vi "Physics_Engine_Core.vi"(0 "Design Constants":T6={"P_amb (psia)"=0.125, "T_in (Deg F)"=14.7, "R_air (ft*lbf)/(lbm*R)"=530.0, "g_c (lbm*ft)/(lbf*s^2)"=53.35, "specific heat ratio"=32.17, "Viscousity (lbm)/(ft*s)"=1.4, "Cd"=0.95, "Mass Flow (lbm/min) vs. Pressure Drop (inH2O) - Real Data"=[[0.5, 0.015], [1.0, 0.062], [1.5, 0.141], [2.0, 0.252], [2.5, 0.395], [3.5, 0.778]]} {"Mass Flow (lbm/min) vs. Pressure Drop (inH2O) - Real Data" format="%_3g"; "P_amb (psia)" format="%#_4g"}, 1 "Calibration Data":T8, 4 "Design Tuners":T7 {"OAR" items=["0.92"=0.92, "0.93"=0.93, "0.94"=0.94, "0.95"=0.95, "0.96"=0.96]; "D_h (in)" items=["0.0625"=0.0625, "0.125"=0.125, "0.250"=0.25]; "Pipe_Diameter (in)" min=0.1 max=6.0 scale=0.0..6.0 scale format="%#_3g"; "Length (in)" min=0.1 max=5.0 scale=0.0..6.0 scale format="%#_3g"; "Outlet Diameter (in)" min=0.1 max=5.0 scale=0.0..5.0 scale format="%#_3g"; "Inlet Diameter (in)" min=0.1 max=5.0 scale=0.0..5.0}, 5 "error in (no error)":errorcluster, 6 "Enum":T5) -> (14 "empirical curve":T3, 15 "total curve":T2, 16 "tap curve":T1, 17 "outcome":cluster{"pass/fail":dbl[], "error_pct":dbl[]}, 18 "parameters_output":T4, 19 "error out":errorcluster)   [LabVIEW 2025, in "Acquisition.lvlib"]
uses:
  Acquisition/Acquisition.lvlib
  controls/Calibration_Data.ctl
  controls/Tuners.ctl
  controls/Constants.ctl
  controls/Mode Enum.ctl
panel:
  out "Re_c":dbl[](array[numeric])
  # "Empirical Flow Path Data"
  # "Mass Flow\n (lbm/min)"
  # "Pressure Drop \n    (inH2O)"
  # "Honeycomb Parameters"
  # "Orifice Parameters"
  # "Pipe Parameters"
  # "AIRFLOW SIMULATOR"
  # "Mass_flowrate"
  # "Pipe_Diameter"
  # "Outlet_Diameter"
  # "Inlet_Diameter"
  # "Honeycomb_Length"
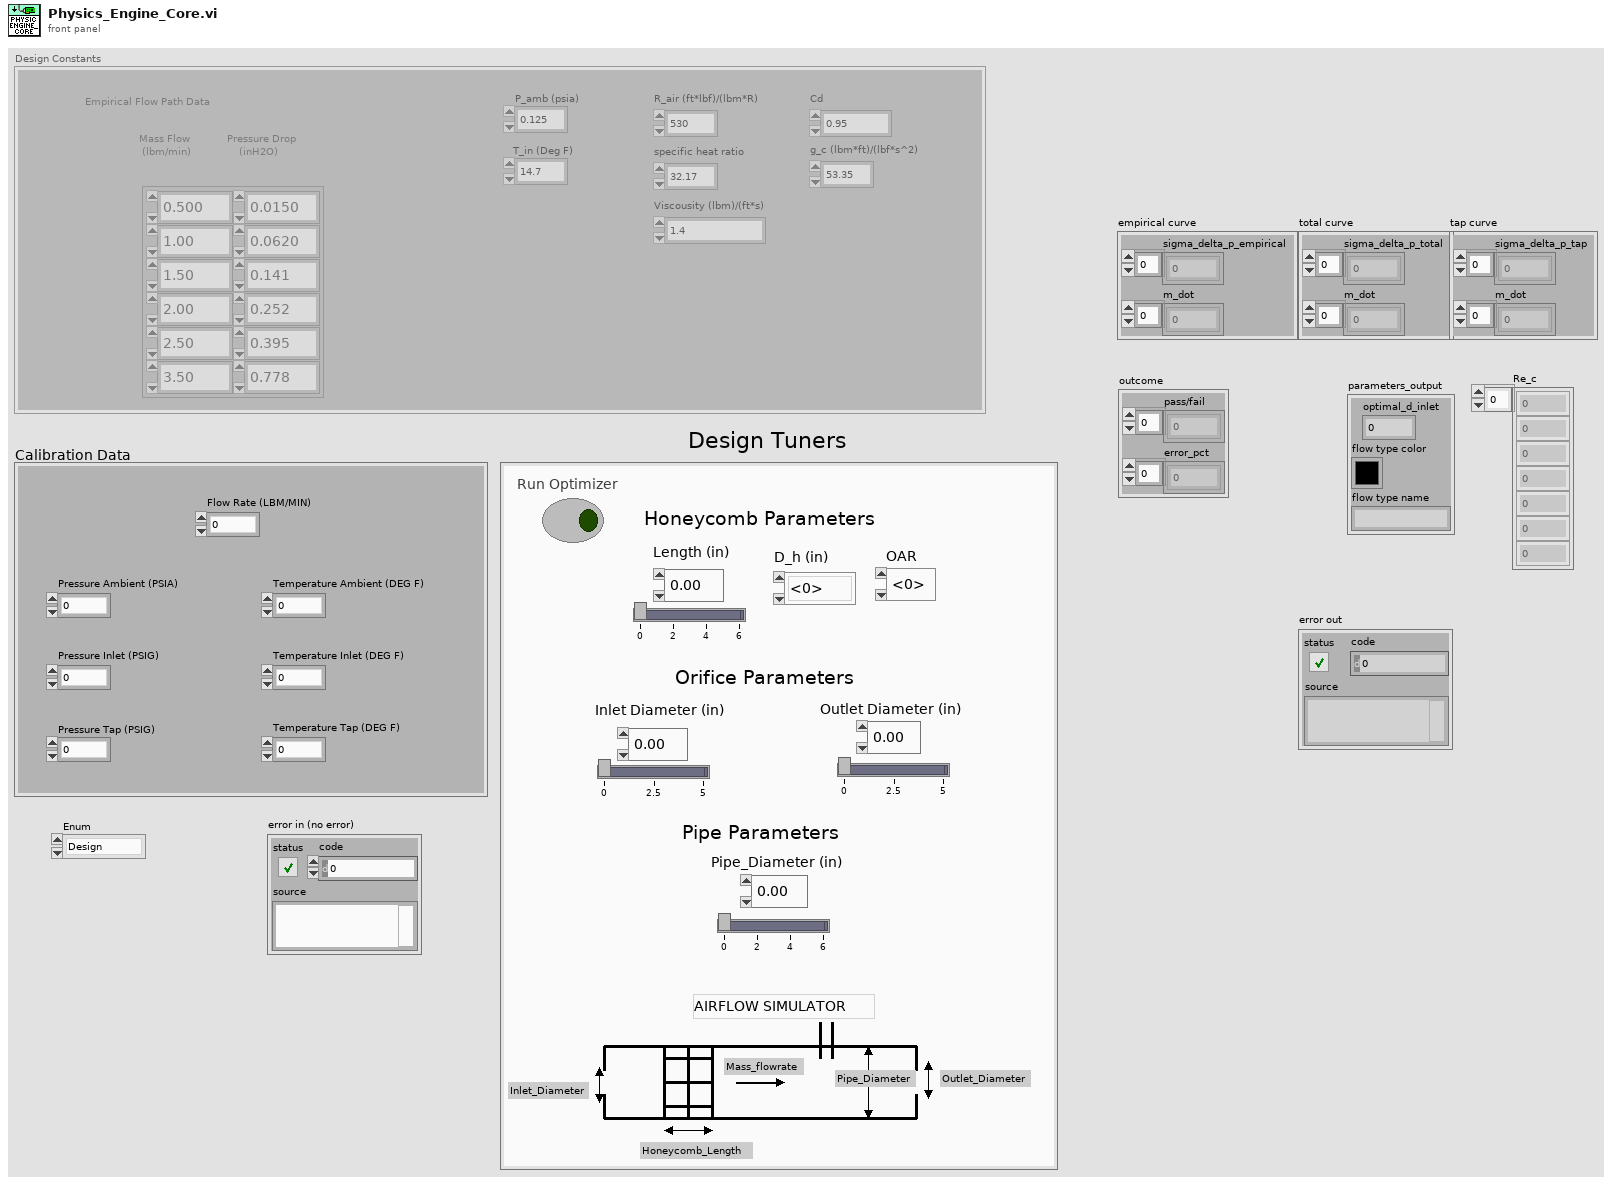
[diagram p1: front panel]
types:
  T1 = cluster{"sigma_delta_p_tap":dbl[], "m_dot":dbl[]}
  T2 = cluster{"sigma_delta_p_total":dbl[], "m_dot":dbl[]}
  T3 = cluster{"sigma_delta_p_empirical":dbl[], "m_dot":dbl[]}
  T4 = cluster{"optimal_d_inlet":dbl, "flow type color":u32, "flow type name":string}
  T5 = typedef "Mode Enum.ctl" = enum16{"Design", "Calibration"}
  T6 = typedef "Constants.ctl" = cluster{"P_amb (psia)":dbl, "T_in (Deg F)":dbl, "R_air (ft*lbf)/(lbm*R)":dbl, "g_c (lbm*ft)/(lbf*s^2)":dbl, "specific heat ratio":dbl, "Viscousity (lbm)/(ft*s)":dbl, "Cd":dbl, "Mass Flow (lbm/min) vs. Pressure Drop (inH2O) - Real Data":dbl[][]}
  T7 = typedef "Tuners.ctl" = cluster{"Inlet Diameter (in)":dbl, "Outlet Diameter (in)":dbl, "Length (in)":dbl, "Pipe_Diameter (in)":dbl, "D_h (in)":dbl, "OAR":dbl, "Run Optimizer":bool}
  T8 = typedef "Calibration_Data.ctl" = cluster{"Flow Rate (LBM/MIN)":dbl, "Pressure Ambient (PSIA)":dbl, "Pressure Inlet (PSIG)":dbl, "Pressure Tap (PSIG)":dbl, "Temperature Ambient (DEG F)":dbl, "Temperature Inlet (DEG F)":dbl, "Temperature Tap (DEG F)":dbl}
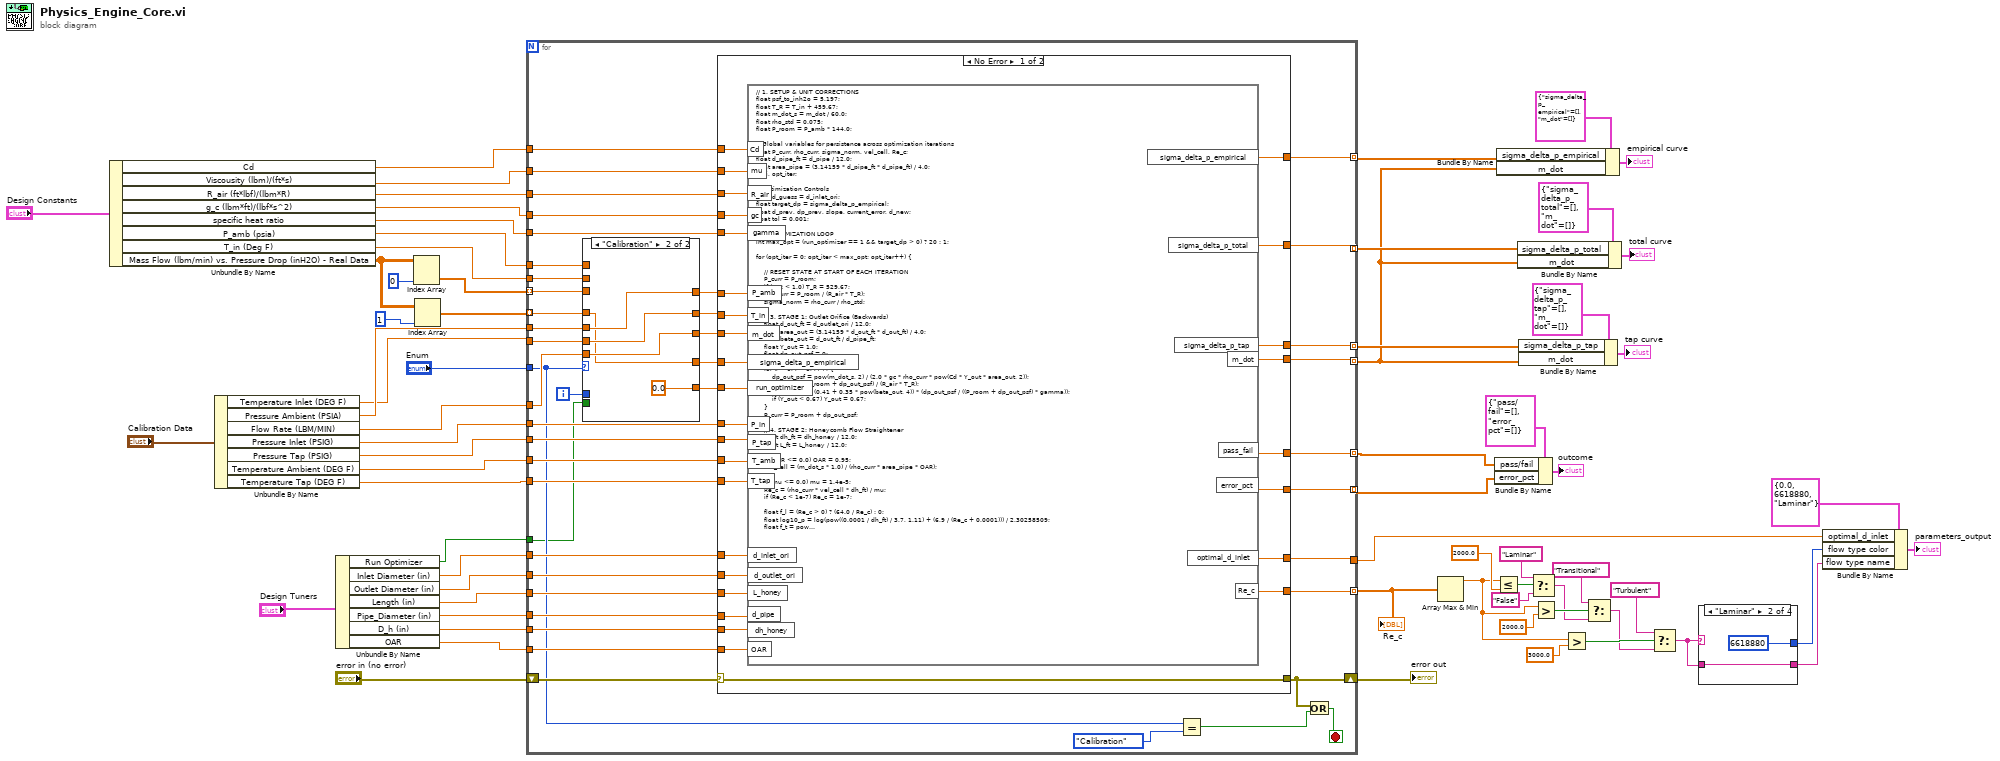
[diagram p0: block diagram]
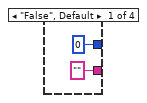
[diagram p2: hidden frame]
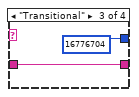
[diagram p3: hidden frame]
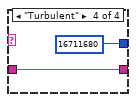
[diagram p4: hidden frame]
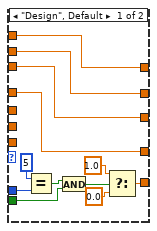
[diagram p5: hidden frame]
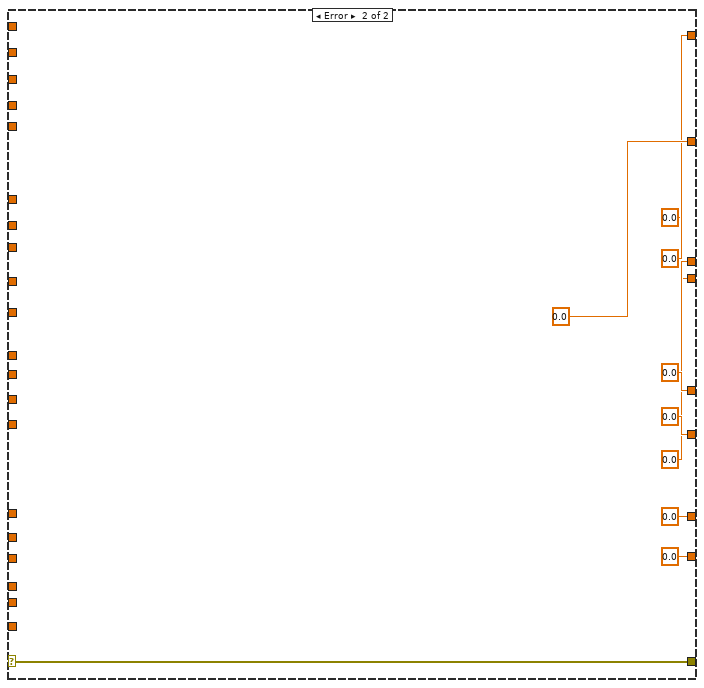
[diagram p6: hidden frame]
diagram:
  n1 = Unbundle By Name("Design Constants") -> ("Cd"=w46:dbl, "Viscousity (lbm)/(ft*s)"=w47:dbl, "R_air (ft*lbf)/(lbm*R)"=w48:dbl, "g_c (lbm*ft)/(lbf*s^2)"=w49:dbl, "specific heat ratio"=w50:dbl, "P_amb (psia)"=w41:dbl, "T_in (Deg F)"=w43:dbl, "Mass Flow (lbm/min) vs. Pressure Drop (inH2O) - Real Data"=w37:dbl[][])
  n2 = Unbundle By Name("Calibration Data") -> ("Temperature Inlet (DEG F)"=w42:dbl, "Pressure Ambient (PSIA)"=w44:dbl, "Flow Rate (LBM/MIN)"=w63:dbl, "Pressure Inlet (PSIG)"=w62:dbl, "Pressure Tap (PSIG)"=w61:dbl, "Temperature Ambient (DEG F)"=w60:dbl, "Temperature Tap (DEG F)"=w59:dbl)
  n3 = Unbundle By Name("Design Tuners") -> ("Run Optimizer"=w35:bool, "Inlet Diameter (in)"=w57:dbl, "Outlet Diameter (in)"=w56:dbl, "Length (in)"=w52:dbl, "Pipe_Diameter (in)"=w53:dbl, "D_h (in)"=w55:dbl, "OAR"=w54:dbl)
  n4 = Index Array(array=w37, index (col)=0) -> (element=w39:dbl[])  [unwired: 1 in]
  n5 = Index Array(array=w37, index (col)=1) -> (element=w36:dbl[])  [unwired: 1 in]
  n6 = for {
    tunnel: w63 -> [w82]
    tunnel: w62 -> [w108]
    tunnel: w61 -> [w107]
    tunnel: w60 -> [w106]
    tunnel: w59 -> [w105]
    tunnel: w57 -> [w104]
    tunnel: w56 -> [w103]
    tunnel: w55 -> [w102]
    tunnel: w54 -> [w101]
    tunnel: w53 -> [w100]
    tunnel: w52 -> [w99]
    tunnel: w50 -> [w98]
    tunnel: w49 -> [w97]
    tunnel: w48 -> [w96]
    tunnel: w47 -> [w95]
    tunnel: w46 -> [w94]
    tunnel: [w93] -> w8 mode=indexing
    shift-right: [w77] -> w65
    shift-left: "error in (no error)" -> [w109]
    tunnel: "Enum" -> [w78]
    tunnel: w44 -> [w92]
    tunnel: w43 -> [w91]
    tunnel: w42 -> [w90]
    tunnel: w41 -> [w89]
    tunnel: w39 -> [w88] mode=indexing
    tunnel: w36 -> [w84] mode=indexing
    tunnel: [w81] -> w11 mode=indexing
    tunnel: [w80] -> w13 mode=indexing
    tunnel: [w74] -> w5 mode=indexing
    tunnel: [w73] -> w19
    tunnel: w35 -> [w70]
    tunnel: [w69] -> w20 mode=indexing
    tunnel: [w68] -> w9 mode=indexing
    tunnel: [w67] -> w4 mode=indexing
    i -> [w72]
    stop <- w75 stop-if-true
    n7 = case shown="\"Calibration\"" w78 {
      tunnel: w92 -> [_ w126]
      tunnel: [w121 w126] -> w87
      tunnel: w91 -> [w120 _]
      tunnel: w90 -> [_ w125]
      tunnel: [w120 w125] -> w86
      tunnel: w89 -> [w121 _]
      tunnel: w88 -> [w119 _]
      tunnel: [w119 w124] -> w85
      tunnel: w84 -> [w118 w123]
      tunnel: [w118 w123] -> w83
      tunnel: w82 -> [_ w124]
      tunnel: w72 -> [w111 _]
      tunnel: [w116 0.0 ("f")] -> w71
      tunnel: w70 -> [w110 _]
      frame "Design", Default {
        n8 = Equal?(x=5 ("y"), y=w111) -> (x = y?=w114:bool)
        n9 = And(x=w114, y=w110) -> (x .and. y?=w113:bool)
        n10 = Select(t=1.0, s=w113, f=0.0) -> (s? t:f=w116:dbl)
      }
      frame "Calibration" {
      }
    }
    n11 = case shown="No Error" w109 {
      selector: w109 -> [w143 w164]
      tunnel: [w143 w164] -> w77
      tunnel: w87 -> [w155 _]
      tunnel: w85 -> [w154 _]
      tunnel: w108 -> [w153 _]
      tunnel: w107 -> [w152 _]
      tunnel: w106 -> [w151 _]
      tunnel: w105 -> [w150 _]
      tunnel: w104 -> [w149 _]
      tunnel: w103 -> [w148 _]
      tunnel: w102 -> [w147 _]
      tunnel: w101 -> [w146 _]
      tunnel: w100 -> [w145 _]
      tunnel: w99 -> [w144 _]
      tunnel: w86 -> [w142 _]
      tunnel: w98 -> [w141 _]
      tunnel: w97 -> [w140 _]
      tunnel: w96 -> [w139 _]
      tunnel: w95 -> [w138 _]
      tunnel: w94 -> [w137 _]
      tunnel: [w136 0.0 ("sigma_delta_p")] -> w93
      tunnel: w83 -> [w135 _]
      tunnel: [w134 0.0 ("pass_fail")] -> w81
      tunnel: [w133 0.0 ("error_pct")] -> w80
      tunnel: [w132 0.0 ("sigma_delta_p_tap")] -> w74
      tunnel: [w131 0.0 ("optimal_d_inlet")] -> w73
      tunnel: w71 -> [w130 _]
      tunnel: [w129 0.0] -> w69
      tunnel: [w128 0.0 ("sigma_delta_p_empirical")] -> w68
      tunnel: [w127 0.0 ("m_dot")] -> w67
      frame No Error {
        n12 = formula code="// 1. SETUP & UNIT CORRECTIONS\nfloat psf_to_inh2o = 5.197;\nfloat T_R = T_in + 459.67;\nfloat m_dot_s = m_dot / 60.0;\nfloat rho_std = 0.075;\nfloat P_room = P_amb * 144.0;\n\n// Global variables for persistence across optimization iterations\nfloat P_curr, rho_curr, sigma_norm, vel_cell, Re_c; \nfloat d_pipe_ft = d_pipe / 12.0;\nfloat area_pipe = (3.14159 * d_pipe_ft * d_pipe_ft) / 4.0;\nint i, opt_iter;\n\n// Optimization Controls\nfloat d_guess = d_inlet_ori;\nfloat target_dp = sigma_delta_p_empirical;\nfloat d_prev, dp_prev, slope, current_error, d_new;\nfloat tol = 0.001; \n\n// 2. OPTIMIZATION LOOP\nint max_opt = (run_optimizer == 1 && target_dp > 0) ? 20 : 1;\n\nfor (opt_iter = 0; opt_iter < max_opt; opt_iter++) {\n    \n    // RESET STATE AT START OF EACH ITERATION\n    P_curr = P_room;\n    if (T_R < 1.0) T_R = 529.67; \n    rho_curr = P_room / (R_air * T_R);\n    sigma_norm = rho_curr / rho_std;\n\n    // 3. STAGE 1: Outlet Orifice (Backwards)\n    float d_out_ft = d_outlet_ori / 12.0;\n    float area_out = (3.14159 * d_out_ft * d_out_ft) / 4.0;\n    float beta_out = d_out_ft / d_pipe_ft;\n    float Y_out = 1.0;\n    float dp_out_psf = 0;\n\n    for (i = 0; i < 8; i++) {\n        dp_out_psf = pow(m_dot_s, 2) / (2.0 * gc * rho_curr * pow(Cd * Y_out * area_out, 2));\n        rho_curr = (P_room + dp_out_psf) / (R_air * T_R);\n        Y_out = 1.0 - (0.41 + 0.35 * pow(beta_out, 4)) * (dp_out_psf / ((P_room + dp_out_psf) * gamma));\n        if (Y_out < 0.67) Y_out = 0.67;\n    }\n    P_curr = P_room + dp_out_psf;\n\n    // 4. STAGE 2: Honeycomb Flow Straightener\n    float dh_ft = dh_honey / 12.0;\n    float L_ft = L_honey / 12.0;\n    \n    if (OAR <= 0.0) OAR = 0.95; \n    vel_cell = (m_dot_s * 1.0) / (rho_curr * area_pipe * OAR);\n\n    if (mu <= 0.0) mu = 1.4e-5;\n    Re_c = (rho_curr * vel_cell * dh_ft) / mu;\n    if (Re_c < 1e-7) Re_c = 1e-7; \n\n    float f_l = (Re_c > 0) ? (64.0 / Re_c) : 0;\n    float log10_p = log(pow((0.0001 / dh_ft) / 3.7, 1.11) + (6.9 / (Re_c + 0.0001))) / 2.30258509;\n    float f_t = pow(1.0 / (-1.8 * log10_p), 2);\n    float f_h = (Re_c < 2000) ? f_l : (Re_c > 3000 ? f_t : (f_l + f_t)/2.0);\n\n    P_curr += f_h * (L_ft / dh_ft) * (rho_curr * vel_cell * vel_cell) / (2.0 * gc);\n    rho_curr = P_curr / (R_air * T_R);\n    \n    // CAPTURE TAP PRESSURE (Tap-to-Exit)\n    sigma_delta_p_tap = ((P_curr - P_room) / psf_to_inh2o) * sigma_norm;\n\n    // 5. STAGE 3: Inlet Orifice (Variable for Optimization)\n    float d_in_ft = d_guess / 12.0;\n    float area_in = (3.14159 * d_in_ft * d_in_ft) / 4.0;\n    float beta_in = d_in_ft / d_pipe_ft;\n    float Y_in = 1.0;\n    float dp_in_psf = 0;\n\n    for (i = 0; i < 8; i++) {\n        dp_in_psf = pow(m_dot_s, 2) / (2.0 * gc * rho_curr * pow(Cd * Y_in * area_in, 2));\n        rho_curr = (P_curr + dp_in_psf) / (R_air * T_R);\n        Y_in = 1.0 - (0.41 + 0.35 * pow(beta_in, 4)) * (dp_in_psf / ((P_curr + dp_in_psf) * gamma));\n        if (Y_in < 0.67) Y_in = 0.67;\n    }\n\n    // 6. TOTAL CALCULATION (Inlet-to-Exit)\n    sigma_delta_p_total = ((P_curr + dp_in_psf - P_room) / psf_to_inh2o) * sigma_norm;\n\n    // OPTIMIZER STEP (Matches Total Pressure to Empirical Target)\n    if (run_optimizer == 1) {\n        current_error = sigma_delta_p_total - target_dp;\n        if (abs(current_error) < tol) break; \n\n        if (opt_iter == 0) {\n            d_prev = d_guess;\n            dp_prev = sigma_delta_p_total;\n            d_guess += (d_guess * 0.01); \n        } else {\n            slope = (sigma_delta_p_total - dp_prev) / (d_guess - d_prev);\n            d_prev = d_guess;\n            dp_prev = sigma_delta_p_total;\n            d_new = d_guess - 0.8 * (current_error / slope);\n            d_guess = d_new;\n        }\n        \n        if (d_guess < 0.2) d_guess = 0.2;\n        if (d_guess > (d_pipe * 0.95)) d_guess = d_pipe * 0.95;\n    }\n}\n\n// 7. FINAL OUTPUTS\noptimal_d_inlet = (d_guess != d_guess) ? d_inlet_ori : d_guess;\n\nif (target_dp != 0) {\n    error_pct = ((sigma_delta_p_total - target_dp) / target_dp) * 100.0;\n} else {\n    error_pct = 0;\n}\n\npass_fail = (abs(error_pct) <= 2.0) ? 1 : 0;"("P_amb"=w155, "m_dot"=w154, "P_in"=w153, "P_tap"=w152, "T_amb"=w151, "T_in"=w142, "T_tap"=w150, "d_inlet_ori"=w149, "d_outlet_ori"=w148, "L_honey"=w144, "dh_honey"=w147, "OAR"=w146, "d_pipe"=w145, "gamma"=w141, "gc"=w140, "R_air"=w139, "mu"=w138, "Cd"=w137, "sigma_delta_p_empirical"=w135, "run_optimizer"=w130) -> ("sigma_delta_p_total"=w136:dbl, "pass_fail"=w134:dbl, "error_pct"=w133:dbl, "sigma_delta_p_tap"=w132:dbl, "optimal_d_inlet"=w131:dbl, "Re_c"=w129:dbl, "sigma_delta_p_empirical"=w128:dbl, "m_dot"=w127:dbl)
      }
      frame Error {
      }
    }
    n13 = Equal?(x=w78, y=Mode_Enum."Calibration" ("Enum 2")) -> (x = y?=w76:bool)
    n14 = Or(x=w77, y=w76) -> (x .or. y?=w75:bool)
  }
  "error out" <- w65
  "Re_c" <- w20
  n15 = Array Max & Min(array=w20) -> (max value=w22:dbl)  [unwired: 3 out]
  n16 = Bundle By Name(cluster=cluster{"pass/fail":dbl[], "error_pct":dbl[]} {"pass/fail"=[], "error_pct"=[]}, "pass/fail"=w11, "error_pct"=w13) -> (→"outcome":cluster{"pass/fail":dbl[], "error_pct":dbl[]})
  n17 = Less Or Equal?(x=w22, y=2000.0) -> (x <= y?=w34:bool)
  n18 = Bundle By Name(cluster=T3 {"sigma_delta_p_empirical"=[], "m_dot"=[]}, "sigma_delta_p_empirical"=w9, "m_dot"=w4) -> (→"empirical curve":T3)
  n19 = Bundle By Name(cluster=T2 {"sigma_delta_p_total"=[], "m_dot"=[]}, "sigma_delta_p_total"=w8, "m_dot"=w4) -> (→"total curve":T2)
  n20 = Bundle By Name(cluster=T1 {"sigma_delta_p_tap"=[], "m_dot"=[]}, "sigma_delta_p_tap"=w5, "m_dot"=w4) -> (→"tap curve":T1)
  n21 = Select(t="Laminar", s=w34, f="False") -> (s? t:f=w29:string)
  n22 = Greater?(x=w22, y=2000.0) -> (0:w30:bool)
  n23 = Greater?(x=w22, y=3000.0) -> (0:w27:bool)
  n24 = Select(t="Transitional", s=w30, f=w29) -> (s? t:f=w25:string)
  n25 = Select(t="Turbulent", s=w27, f=w25) -> (s? t:f=w21:string)
  n26 = case shown="\"Laminar\"" w21 {
    tunnel: [u32 0 u32 6618880 u32 16776704 u32 16711680] -> w18
    tunnel: ["" ("f") w167 w169 w171] -> w16
    tunnel: w21 -> [_ w167 w169 w171]
    frame "False", Default {
    }
    frame "Laminar" {
    }
    frame "Transitional" {
    }
    frame "Turbulent" {
    }
  }
  n27 = Bundle By Name(cluster=T4 {"optimal_d_inlet"=0.0, "flow type color"=6618880, "flow type name"="Laminar"} ("input cluster"), "optimal_d_inlet"=w19, "flow type color"=w18, "flow type name"=w16) -> (→"parameters_output":T4)
